vi "Handle Messages.vi"(8 "error in (no error)":errorcluster, 9 "Message Data":variant, 10 "Message":string, 11 "Process In":refnum<class "Debug Process.lvclass">) -> (0 "error out":errorcluster, 3 "Process Out":refnum<class "Debug Process.lvclass">)   [LabVIEW 2020, in "Debug Process.lvclass"]
doc: "This is the core VI handling incomming messages to the process. This VI should be overridden to add functionality to the process or override functionality implemented by a parent. Any message not handled should be sent to the parent method using the default case. \nEach state should be atomic and states should in general avoid enqueueing new messages from within this method, as there might be other messages interleaved in the queue from the outside. For cyclic iteration of an action, using a Helper Loop is recommended."
uses:
  Debug Process.lvclass
  Public/Lifecycle/Lifecycle State.ctl
  Debug Process.lvclass/Debug Process.ctl
  Public/Lifecycle/Leave Process Loop.vi
  <vilib>/Utility/error.llb/Clear Errors.vi
  Public/Read Name.vi
  <vilib>/Utility/error.llb/Error Cluster From Error Code.vi
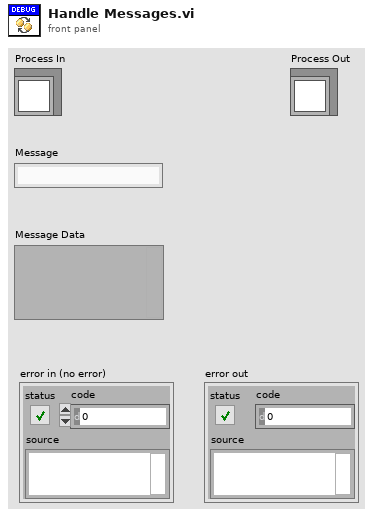
[diagram p1: front panel]
types:
  T1 = typedef "Debug Process.lvclass/Lifecycle State.ctl" = enum16{"Uninitialized", "Initialized", "Started", "Running", "Stopped", "Finished"}
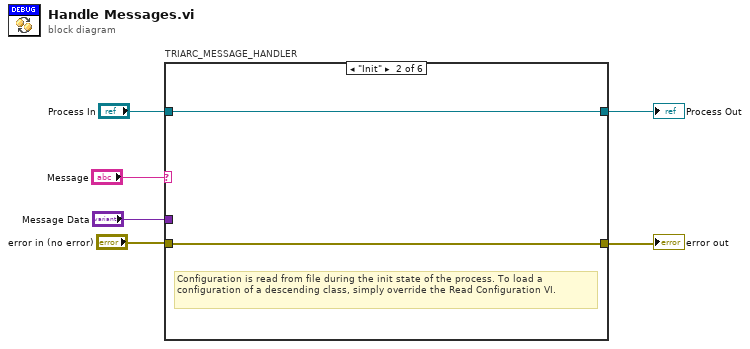
[diagram p0: block diagram]
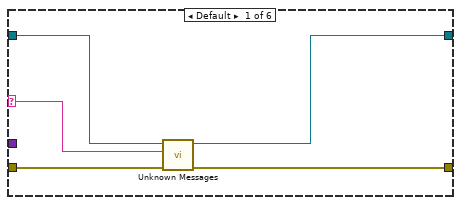
[diagram p2: hidden frame]
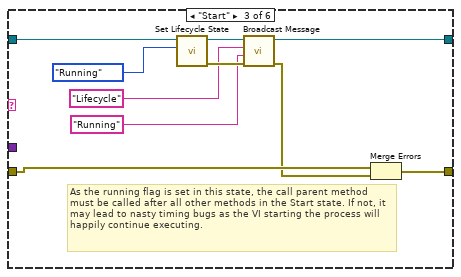
[diagram p3: hidden frame]
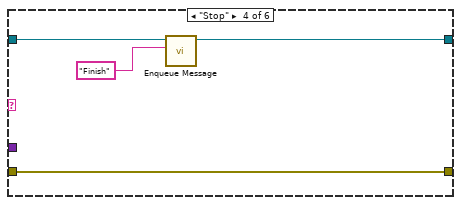
[diagram p4: hidden frame]
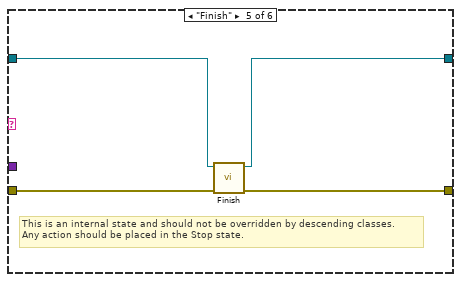
[diagram p5: hidden frame]
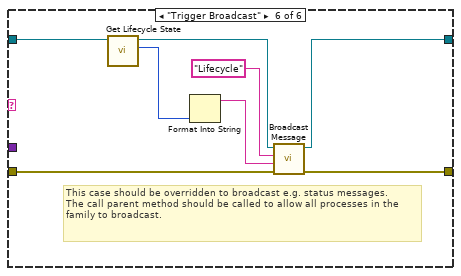
[diagram p6: hidden frame]
diagram:
  n1 = case "TRIARC_MESSAGE_HANDLER" shown="\"Init\"" "Message" {
    selector: "Message" -> [w11 _ _ _ _ _]
    tunnel: [w8 w12 w22 w25 w31 w35] -> w5
    tunnel: "error in (no error)" -> [w7 w12 w21 w25 w30 w32]
    tunnel: [w10 w13 w14 w24 w28 w39] -> w3
    tunnel: "Process In" -> [w9 w13 w23 w26 w29 w38]
    tunnel: "Message Data" -> [_ _ _ _ _ _]
    frame Default {
      n2 = call "Unknown Messages.vi"("error in (no error)"=w7, "Message"=w11, "Process In"=w9) -> ("error out"=w8:errorcluster, "Process Out"=w10:refnum<class "Debug Process.lvclass">)  [unwired: 7 in]
    }
    frame "Init" {
      # "Configuration is read from file during the init state of the process. To load a configuration of a descending class, simply override the Read Configuration VI."
    }
    frame "Start" {
      # "As the running flag is set in this state, the call parent method must be called after all other methods in the Start state. If not, it may lead to nasty timing bugs as the VI starting the process will happily continue executing."
      n3 = call "Set Lifecycle State.vi"("Lifecycle State"=Lifecycle_State."Running", "Process In"=w23) -> ("error out"=w19:errorcluster, "Process Out"=w20:refnum<class "Debug Process.lvclass">)  [unwired: 8 in]
      n4 = call-dynamic "Broadcast Message.vi"("error in (no error)"=w19, "Message Data"="Running" ("Message"), "Message"="Lifecycle", "Process In"=w20) -> ("error out"=w18:errorcluster, "Process Out"=w14:refnum<class "Debug Process.lvclass">)  [unwired: 6 in]
      n5 = Merge Errors(w21, w18) -> (w22:errorcluster)
    }
    frame "Stop" {
      n6 = call "Enqueue Message.vi"("Message"="Finish", "Process In"=w26) -> ("Process Out"=w24:refnum<class "Debug Process.lvclass">)  [unwired: 8 in, 1 out]
    }
    frame "Finish" {
      # "This is an internal state and should not be overridden by descending classes.\nAny action should be placed in the Stop state."
      n7 = call "Finish.vi"("error in (no error)"=w30, "Process In"=w29) -> ("error out"=w31:errorcluster, "Process Out"=w28:refnum<class "Debug Process.lvclass">)  [unwired: 8 in]
    }
    frame "Trigger Broadcast" {
      # "This case should be overridden to broadcast e.g. status messages.\nThe call parent method should be called to allow all processes in the family to broadcast."
      n8 = call "Get Lifecycle State.vi"("Process In"=w38) -> ("Lifecycle State"=w34:T1, "Process Out"=w36:refnum<class "Debug Process.lvclass">)  [unwired: 7 in, 2 out]
      n9 = Format Into String(w34) -> (resulting string=w33:string)  [unwired: 3 in, 1 out]
      n10 = call-dynamic "Broadcast Message.vi"("error in (no error)"=w32, "Message Data"=w33, "Message"="Lifecycle", "Process In"=w36) -> ("error out"=w35:errorcluster, "Process Out"=w39:refnum<class "Debug Process.lvclass">)  [unwired: 6 in]
    }
  }
  "error out" <- w5
  "Process Out" <- w3
